vi "PRIVATE.ProcCases.vi"(0 "i ref in":refnum<vi>, 1 "selector":string, 3 "call cluster":T2={"Object"="", "Selector"="", "CallType"=enum."synchronous", "Async Object"="", "Async Selector"="", "Data Descriptor"="", "Data"=[], "Error #"=0, "Expire"=0}, 5 "error in (no error)":errorcluster) -> (14 "i ref out":refnum<vi>, 17 "answer cluster":T2={"Object"="", "Selector"="", "CallType"=enum."synchronous", "Async Object"="", "Async Selector"="", "Data Descriptor"="", "Data"=[], "Error #"=0, "Expire"=0}, 19 "error out":errorcluster)   [LabVIEW 2012, in "MrClean.lvlib"]
doc: "This method is called by a process from within the default case in the event loop. The methods of a class that are linked to events will be called from THIS method. Add your code here."
uses:
  MrClean.lvlib
  CSCore/CSSystem/CoreLib/CoreLib.lvlib
  CSCore/BaseProcess/BaseProcess.lvlib
  CSCore/CSSystem/CoreLib/CoreLib.string 2 byte array.vi
  CSCore/CSSystem/CoreLib/CoreLib.byte array 2 double.vi
  CSCore/CSSystem/CoreDefs/CoreDefs.call_type.ctl
  CSCore/BaseProcess/BaseProcess.descriptor string definition.ctl
  CSCore/CSSystem/CoreDefs/CoreDefs.rawDataType.ctl
panel:
  in  "Data":T1
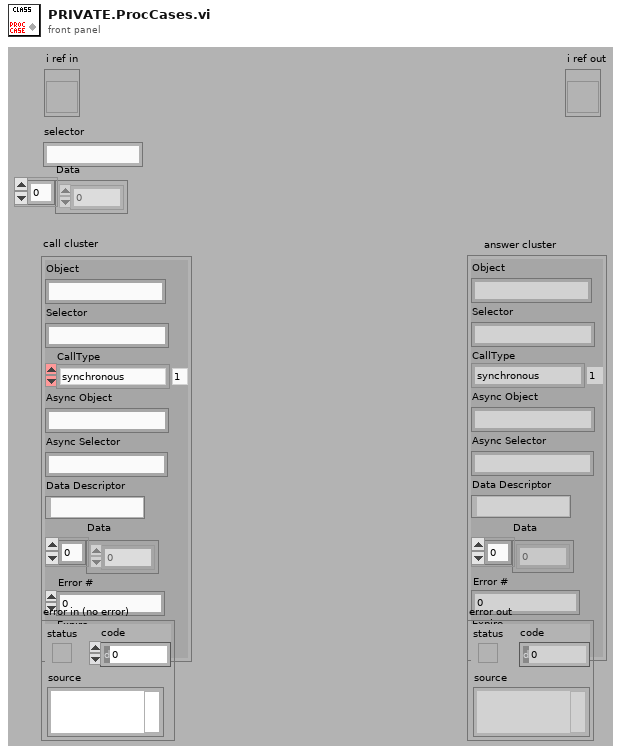
[diagram p1: front panel]
types:
  T1 = typedef "CoreDefs.rawDataType.ctl" = i8[]
  T2 = typedef "CoreDefs.call_type.ctl" = cluster{"Object":string, "Selector":string, "CallType":enum16{"simple", "synchronous", "asynchronous"}, "Async Object":string, "Async Selector":string, "Data Descriptor":T3, "Data":T1, "Error #":i32, "Expire":u32}
  T3 = typedef "BaseProcess.lvlib/BaseProcess.descriptor string definition.ctl" = string
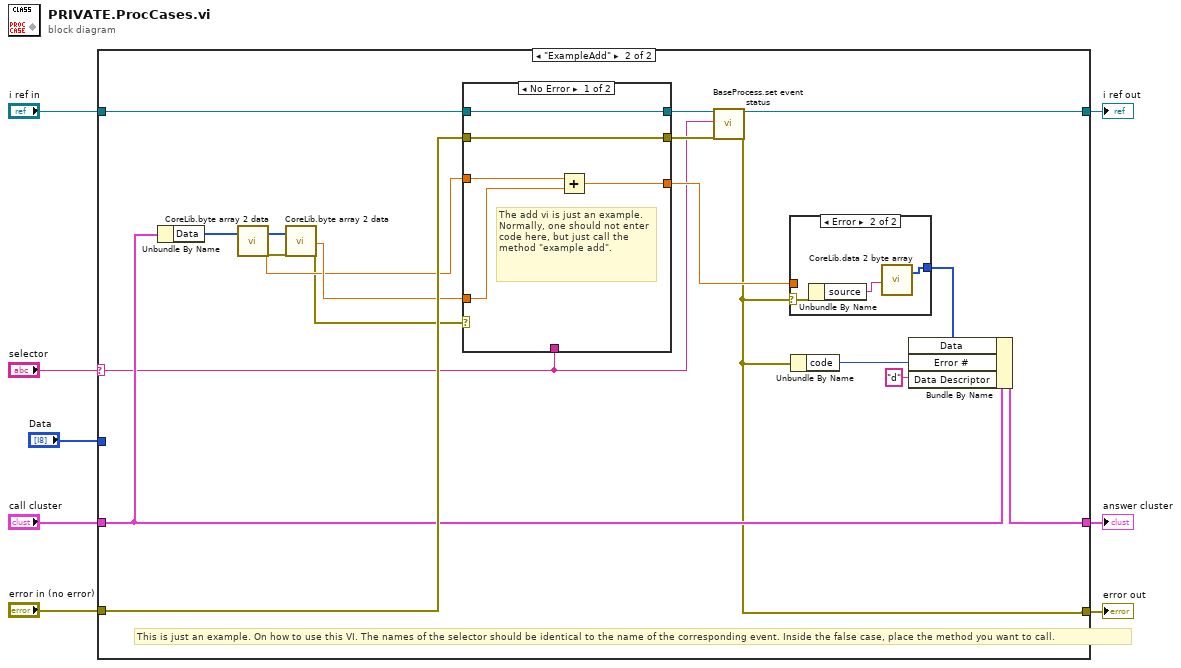
[diagram p0: block diagram]
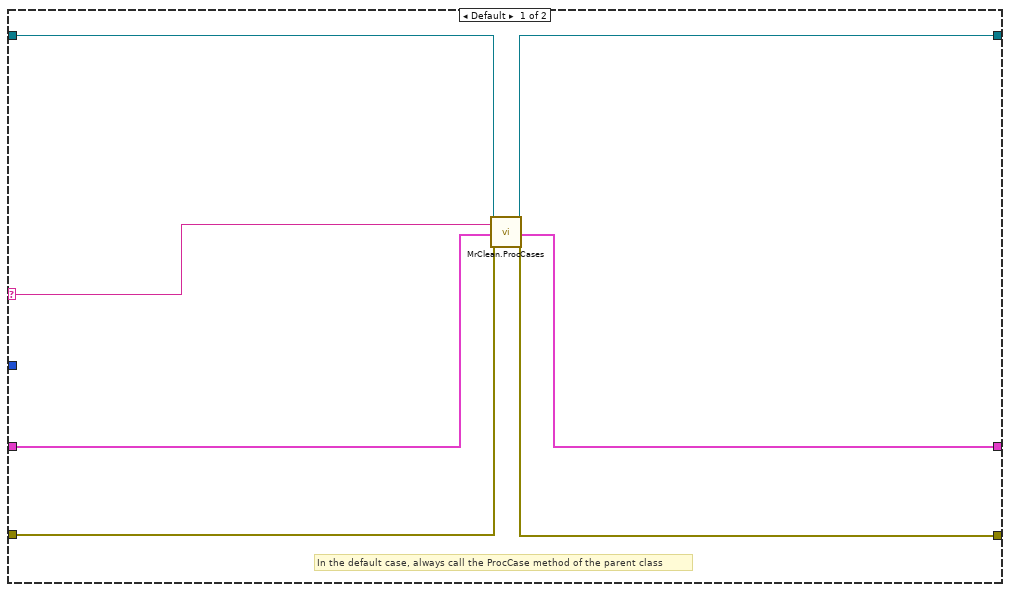
[diagram p2: hidden frame]
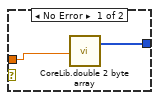
[diagram p3: hidden frame]
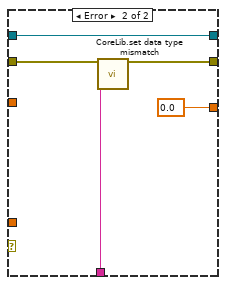
[diagram p4: hidden frame]
diagram:
  n1 = case shown="\"ExampleAdd\"" "selector" {
    selector: "selector" -> [w10 w25]
    tunnel: "Data" -> [_ _]
    tunnel: "i ref in" -> [w9 w34]
    tunnel: [w15 w24] -> w4
    tunnel: "call cluster" -> [w11 w30]
    tunnel: [w12 w29] -> w7
    tunnel: "error in (no error)" -> [w14 w33]
    tunnel: [w13 w26] -> w2
    frame Default {
      # "In the default case, always call the ProcCase method of the parent class"
      n2 = call "MrClean.ProcCases.vi"("i ref in"=w9, "selector"=w10, "call cluster"=w11, "error in (no error)"=w14) -> ("i ref out"=w15:refnum<vi>, "answer cluster"=w12:T2, "error out"=w13:errorcluster)  [unwired: 13 in]
    }
    frame "ExampleAdd" {
      # "This is just an example. On how to use this VI. The names of the selector should be identical to the name of the corresponding event. Inside the false case, place the method you want to call."
      n3 = Unbundle By Name(w30) -> ("Data"=w21:T1)
      n4 = call-poly "CoreLib.byte array 2 data.vi"("byteArray"=w21) -> ("byteArray out"=w20:T1, "d64"=w17:dbl, "error out"=w19:errorcluster)  [unwired: 16 in]
      n5 = call-poly "CoreLib.byte array 2 data.vi"("byteArray"=w20, "error in (no error)"=w19) -> ("d64"=w18:dbl, "error out"=w16:errorcluster)  [unwired: 15 in, 1 out]
      n6 = case shown="No Error" w16 {
        tunnel: [w41 w49] -> w28
        tunnel: w34 -> [w41 w49]
        tunnel: w33 -> [w42 w48]
        tunnel: [w42 w47] -> w27
        tunnel: w18 -> [w44 _]
        tunnel: [w43 0.0] -> w32
        tunnel: w25 -> [_ w45]
        tunnel: w17 -> [w40 _]
        frame No Error {
          # "The add vi is just an example. Normally, one should not enter code here, but just call the method \"example add\"."
          n7 = Add(x=w40, y=w44) -> (x+y=w43:dbl)
        }
        frame Error {
          n8 = call "CoreLib.set data type mismatch.vi"("error in (no error)"=w48, "error source"=w45) -> ("error out"=w47:errorcluster)  [unwired: 17 in]
        }
      }
      n9 = call "BaseProcess.set event status.vi"("i ref in"=w28, "EventStatus"=w25, "error in (no error)"=w27) -> ("i ref out"=w24:refnum<vi>, "error out"=w26:errorcluster)  [unwired: 14 in, 1 out]
      n10 = case shown="Error" w26 {
        selector: w26 -> [_ w39]
        tunnel: w32 -> [w36 _]
        tunnel: [w35 w37] -> w22
        frame No Error {
          n11 = call "CoreLib.double 2 byte array.vi"("f64"=w36) -> ("byteArray out"=w35:T1)  [unwired: 18 in]
        }
        frame Error {
          n12 = Unbundle By Name(w39) -> ("source"=w38:string)
          n13 = call-poly "CoreLib.data 2 byte array.vi"("string"=w38) -> ("byteArray out"=w37:T1)  [unwired: 18 in]
        }
      }
      n14 = Unbundle By Name(w26) -> ("code"=w31:i32)
      n15 = Bundle By Name(cluster=w30, "Data"=w22, "Error #"=w31, "Data Descriptor"="d") -> (w29:T2)
    }
  }
  "answer cluster" <- w7
  "i ref out" <- w4
  "error out" <- w2
